vi "Emballage_BDD_GVF_Param_produit.vi"(6 "Produit_Formate IN":string, 8 "Error in":errorcluster caption="Error in (no error)", 9 "Produit IN":string, 10 "Tableau param produit":string[](array[string]), 11 "Énum":enum16{"set", "get"}(ring)=enum."get") -> (0 "Error out":errorcluster, 2 "Produit OUT":string, 3 "CLS_param_produit":T1, 4 "Produit_Formate OUT":string)   [LabVIEW 2020]
uses:
  Emballage_BDD_param_Produit.ctl
panel:
  out "ID":string
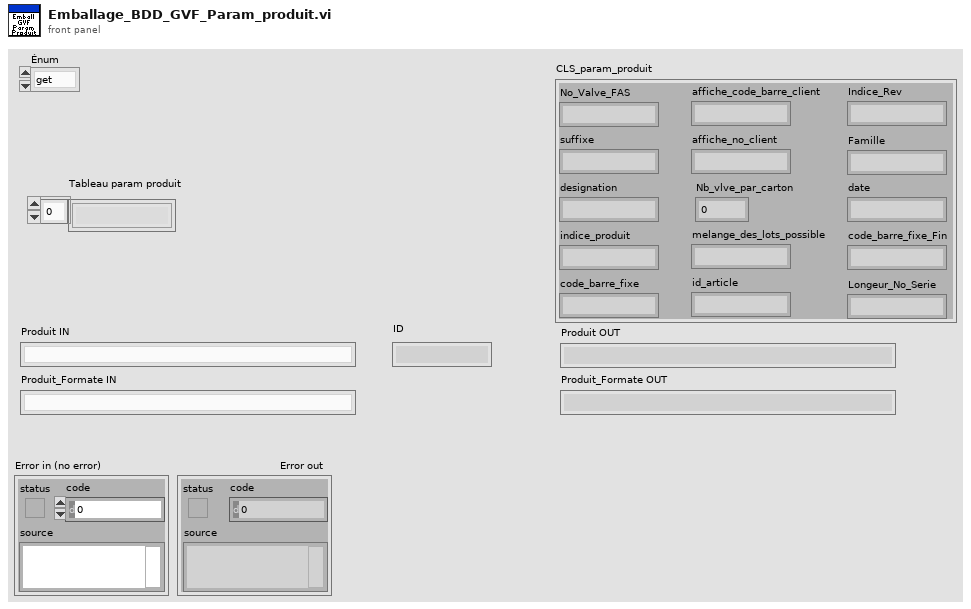
[diagram p1: front panel]
types:
  T1 = typedef "Emballage_BDD_param_Produit.ctl" = cluster{"No_Valve_FAS":string, "suffixe":string, "designation":string, "indice_produit":string, "code_barre_fixe":string, "affiche_code_barre_client":string, "affiche_no_client":string, "Nb_vlve_par_carton":u16, "melange_des_lots_possible":string, "id_article":string, "Indice_Rev":string, "Famille":string, "date":string, "code_barre_fixe_Fin":string, "Longeur_No_Serie":string}
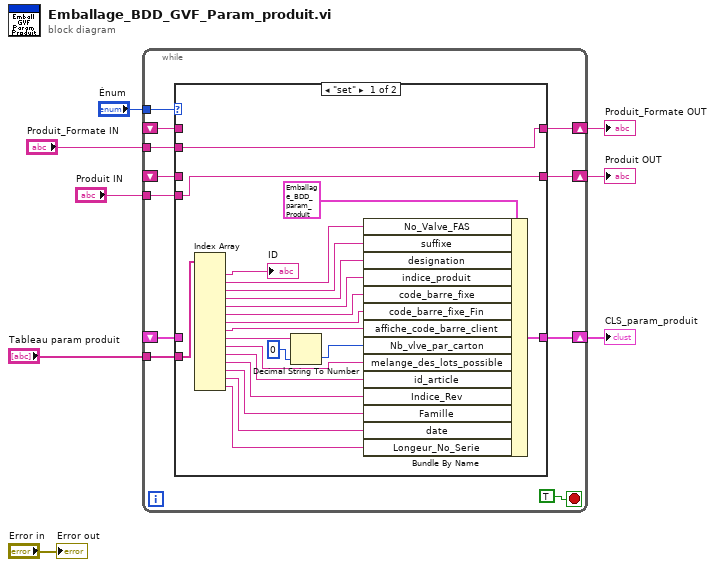
[diagram p0: block diagram]
diagram:
  n1 = while {
    tunnel: "Énum" -> [w18]
    shift-right: [w14] -> w7
    shift-left: _ -> [w13]
    shift-right: [w17] -> w6
    shift-left: _ -> [w15]
    tunnel: "Produit IN" -> [w16]
    tunnel: "Tableau param produit" -> [w12]
    tunnel: "Produit_Formate IN" -> [w10]
    shift-right: [w11] -> w2
    shift-left: _ -> [w9]
    stop <- TRUE stop-if-true
    n2 = case shown="\"set\"" w18 {
      tunnel: [w41 w44] -> w17
      tunnel: w16 -> [w41 _]
      tunnel: w15 -> [_ w44]
      tunnel: [w39 w43] -> w14
      tunnel: w13 -> [_ w43]
      tunnel: w12 -> [w38 _]
      tunnel: [w20 w42] -> w11
      tunnel: w10 -> [w20 _]
      tunnel: w9 -> [_ w42]
      frame "set" {
        n3 = Index Array(array=w38) -> (element #1=→"ID":string, element #2=w37:string, element #3=w36:string, element #4=w35:string, element #5=w34:string, element #6=w33:string, element #7=w28:string, element #8=w29:string, element #9=w27:string, element #10=w26:string, element #11=w25:string, element #12=w24:string, element #13=w23:string, element #14=w22:string, element #15=w21:string)  [unwired: 15 in]
        n4 = Decimal String To Number(string=w27, default (0L)=u16 0 ("valeur par défaut (0 I32)")) -> (number=w30:u16)  [unwired: 1 in, 1 out]
        n5 = Bundle By Name(cluster=T1 {"No_Valve_FAS"="", "suffixe"="", "designation"="", "indice_produit"="", "code_barre_fixe"="", "affiche_code_barre_client"="", "affiche_no_client"="", "Nb_vlve_par_carton"=0, "melange_des_lots_possible"="", "id_article"="", "Indice_Rev"="", "Famille"="", "date"="", "code_barre_fixe_Fin"="", "Longeur_No_Serie"=""} ("CLS_param_produit"), "No_Valve_FAS"=w37, "suffixe"=w36, "designation"=w35, "indice_produit"=w34, "code_barre_fixe"=w33, "code_barre_fixe_Fin"=w28, "affiche_code_barre_client"=w29, "Nb_vlve_par_carton"=w30, "melange_des_lots_possible"=w26, "id_article"=w25, "Indice_Rev"=w24, "Famille"=w23, "date"=w22, "Longeur_No_Serie"=w21) -> (w39:T1)
      }
      frame "get", Default {
      }
    }
  }
  "CLS_param_produit" <- w7
  "Produit OUT" <- w6
  "Produit_Formate OUT" <- w2
  "Error out" <- "Error in"
